vi "2-2-1 Flatten to JSON.vi"() -> ()   [LabVIEW 2020]
panel:
  out "JSON string":string
  in  "sensor_data":T1={"temperature"=82.3, "pressure"=1.103, "motor_on"=FALSE, "status"="RUNNING", "timestamp"="2026-07-26 14:32:05"}
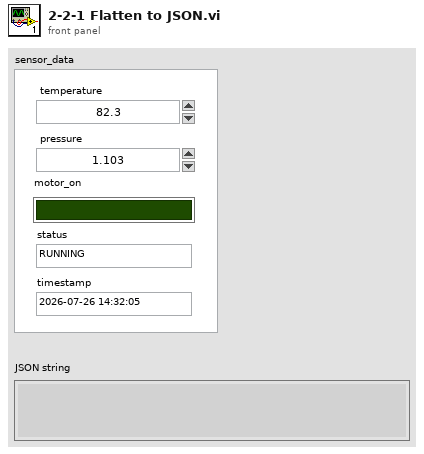
[diagram p1: front panel]
types:
  T1 = cluster{"temperature":dbl, "pressure":dbl, "motor_on":bool, "status":string, "timestamp":string}
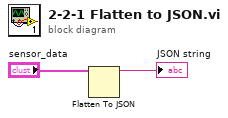
[diagram p0: block diagram]
diagram:
  n1 = Flatten To JSON(anything="sensor_data") -> (JSON string=→"JSON string":string)  [unwired: 2 in, 1 out]
